vi "MFP assistant - KH switcher.vi"(10 "Input array - Differential channels (1 to 8)":dbl[](array[numeric]), 11 "KH setting":T7(ring)) -> ()   [LabVIEW 2016]
uses:
  <userlib>/LevyLab/Krohn Hite 7008/typedefs/KH_control_array.ctl
  <userlib>/LevyLab/Krohn Hite 7008/typedefs/KH_control.ctl
  <userlib>/LevyLab/Krohn Hite 7008/typedefs/Channel-Enum.ctl
  <userlib>/LevyLab/Krohn Hite 7008/typedefs/Gain-Enum.ctl
  <userlib>/LevyLab/Krohn Hite 7008/typedefs/Shunt-Enum.ctl
  <userlib>/LevyLab/Krohn Hite 7008/typedefs/Measure-Enum.ctl
panel:
  in  "Channel Setting":T1=[{"Channel"=enum."Channel 1", "Gain"=enum."10x", "Shunt Resistor"=enum."50k Ohms", "Measure"=enum."Differential"}, {"Channel"=enum."Channel 2", "Gain"=enum."10x", "Shunt Resistor"=enum."Open", "Measure"=enum."Single End (+)"}, {"Channel"=enum."Channel 3", "Gain"=enum."10x", "Shunt Resistor"=enum."50k Ohms", "Measure"=enum."Differential"}, {"Channel"=enum."Channel 4", "Gain"=enum."10x", "Shunt Resistor"=enum."50k Ohms", "Measure"=enum."Differential"}, {"Channel"=enum."Channel 5", "Gain"=enum."10x", "Shunt Resistor"=enum."Open", "Measure"=enum."Single End (+)"}, {"Channel"=enum."Channel 6", "Gain"=enum."10x", "Shunt Resistor"=enum."Open", "Measure"=enum."Single End (+)"}, {"Channel"=enum."Channel 7", "Gain"=enum."10x", "Shunt Resistor"=enum."Open", "Measure"=enum."Single End (+)"}, {"Channel"=enum."Channel 8", "Gain"=enum."10x", "Shunt Resistor"=enum."Open", "Measure"=enum."Single End (+)"}]
  in  "Change KH settings":bool
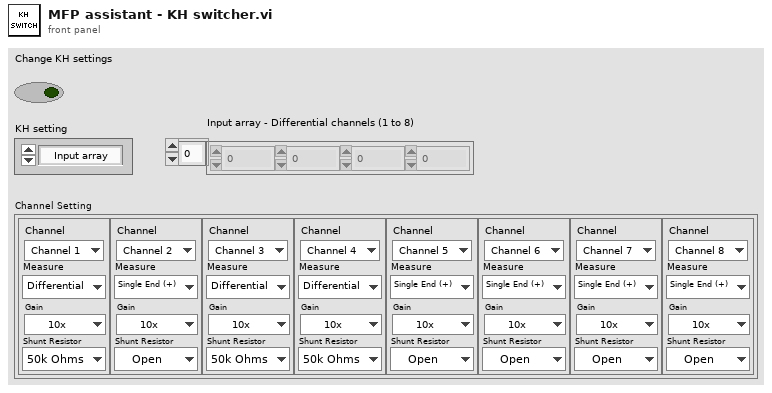
[diagram p1: front panel]
types:
  T1 = typedef "KH_control_array.ctl" = T2[]
  T2 = typedef "KH_control.ctl" = cluster{"Channel":T3, "Gain":T4, "Shunt Resistor":T5, "Measure":T6}
  T3 = typedef "Channel-Enum.ctl" = enum16{"Channel 1", "Channel 2", "Channel 3", "Channel 4", "Channel 5", "Channel 6", "Channel 7", "Channel 8"}
  T4 = typedef "Gain-Enum.ctl" = enum16{"1x", "10x", "100x", "1000x"}
  T5 = typedef "Shunt-Enum.ctl" = enum16{"Open", "50 Ohms", "500 Ohms", "5k Ohms", "50k Ohms"}
  T6 = typedef "Measure-Enum.ctl" = enum16{"Ground", "Differential", "Single End (+)"}
  T7 = enum16{"Input array", "Manual", "All single-end", "All differential"}
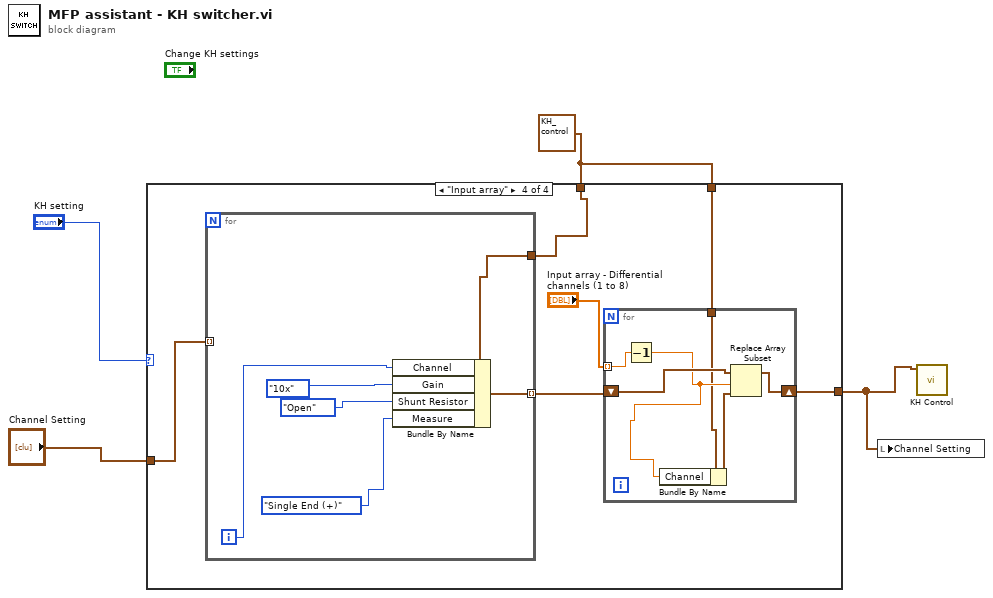
[diagram p0: block diagram]
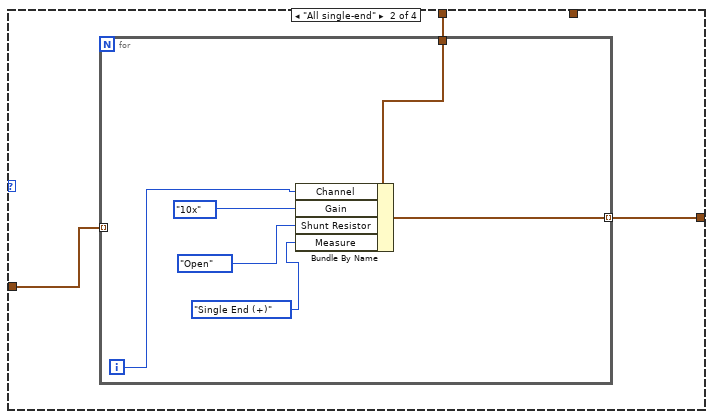
[diagram p3: hidden frame]
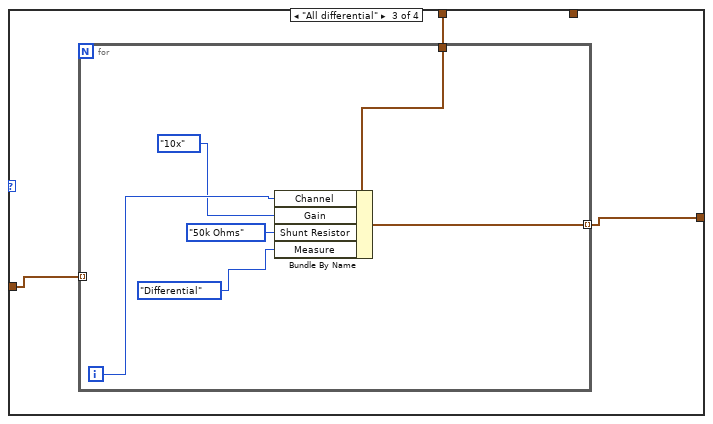
[diagram p4: hidden frame]
diagram:
  w2 = T2 {"Channel"=enum."Channel 1", "Gain"=enum."10x", "Shunt Resistor"=enum."50k Ohms", "Measure"=enum."Differential"} ("System Cluster")
  n1 = case shown="\"Input array\"" "KH setting" {
    tunnel: "Channel Setting" -> [w5 w8 w17 w29]
    tunnel: [w5 w7 w16 w26] -> w1
    tunnel: w2 -> [_ w6 w15 w25]
    tunnel: w2 -> [_ _ _ w24]
    frame "Manual", Default {
    }
    frame "All single-end" {
      n2 = for {
        tunnel: w8 -> [_] mode=indexing
        tunnel: [w13] -> w7 mode=indexing
        tunnel: w6 -> [w12]
        i -> [w14]
        n3 = Bundle By Name(cluster=w12, "Channel"=w14, "Gain"=Gain-Enum."10x", "Shunt Resistor"=Shunt-Enum."Open", "Measure"=Measure-Enum."Single End (+)") -> (w13:T2)
      }
    }
    frame "All differential" {
      n4 = for {
        tunnel: [w22] -> w16 mode=indexing
        tunnel: w17 -> [_] mode=indexing
        tunnel: w15 -> [w21]
        i -> [w23]
        n5 = Bundle By Name(cluster=w21, "Channel"=w23, "Gain"=Gain-Enum."10x", "Shunt Resistor"=Shunt-Enum."50k Ohms", "Measure"=Measure-Enum."Differential") -> (w22:T2)
      }
    }
    frame "Input array" {
      n6 = for {
        tunnel: [w40] -> w28 mode=indexing
        tunnel: w29 -> [_] mode=indexing
        tunnel: w25 -> [w39]
        i -> [w41]
        n7 = Bundle By Name(cluster=w39, "Channel"=w41, "Gain"=Gain-Enum."10x", "Shunt Resistor"=Shunt-Enum."Open", "Measure"=Measure-Enum."Single End (+)") -> (w40:T2)
      }
      n8 = for {
        tunnel: "Input array - Differential channels (1 to 8)" -> [w34] mode=indexing
        shift-right: [w32] -> w26
        shift-left: w28 -> [w35]
        tunnel: w24 -> [w30]
        n9 = Decrement(x=w34) -> (x-1=w31:dbl)
        n10 = Bundle By Name(cluster=w30, "Channel"=w31) -> (w33:T2)
        n11 = Replace Array Subset(array=w35, new element=w33, index=w31) -> (w32:T2[])
      }
    }
  }
  n12 = local write "Channel Setting"(w1) -> ()
  n13 = call <userlib>:"KH Control.vi"("Channel Setting"=w1) -> ()  [unwired: 10 in, 1 out]
